vi "App Stop.vi"(8 "error in (no error)":errorcluster, 10 "Core APIs":T1, 11 "DemoApp in":refnum<class "DemoApp.lvclass">) -> (0 "error out":errorcluster, 3 "DemoApp out":refnum<class "DemoApp.lvclass">)   [LabVIEW 2020, in "VolatusDemo.lvlib" / "DemoApp.lvclass"]
uses:
  DemoApp.lvclass
  Volatus/Core APIs.ctl
  Volatus/VolatusAPI/VolatusAPI.lvclass
  Volatus/Event API/EventAPI.lvclass
  DemoApp.lvclass/DemoApp.ctl
  Volatus/Volatus.lvlib
  Volatus/TelemetryAPI/TelemetryAPI.lvclass
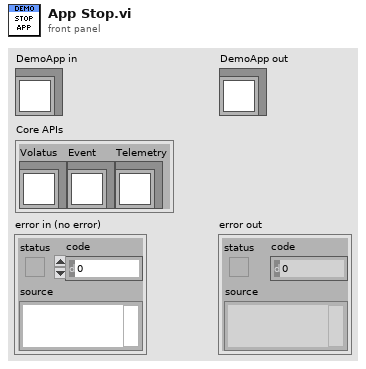
[diagram p1: front panel]
types:
  T1 = typedef "Volatus.lvlib/Core APIs.ctl" = cluster{"Volatus":refnum<class "VolatusAPI.lvclass">, "Event":refnum<class "EventAPI.lvclass">, "Telemetry":refnum<class "TelemetryAPI.lvclass">}
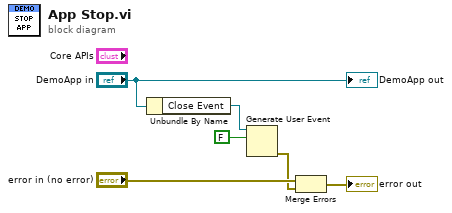
[diagram p0: block diagram]
diagram:
  n1 = Unbundle By Name("DemoApp in") -> ("Close Event"=w4:refnum<user-event>)
  n2 = Generate User Event(user event=w4, event data cluster=FALSE ("event data")) -> (error out=w1:errorcluster)  [unwired: 2 in, 1 out]
  n3 = Merge Errors("error in (no error)", w1) -> (→"error out":errorcluster)
  "DemoApp out" <- "DemoApp in"
